vi "BRig_Host_comm_tcp_parseCmd__getType_v2.vi"(0 "input_strCmd":string, 2 "input_countCmd":i32) -> (14 "output_strType":u8)   [LabVIEW 2014]
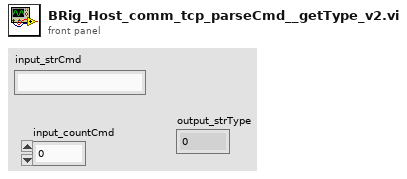
[diagram p1: front panel]
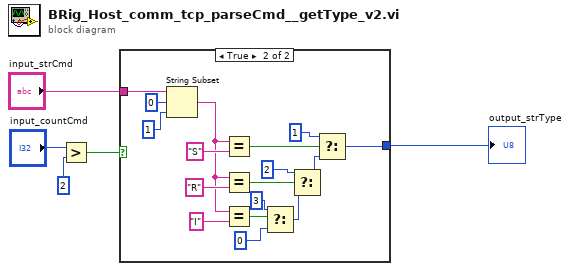
[diagram p0: block diagram]
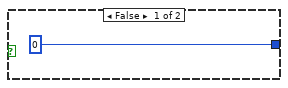
[diagram p2: hidden frame]
diagram:
  n1 = Greater?(x="input_countCmd", y=2) -> (0:w3:bool)
  n2 = case shown="True" w3 {
    tunnel: "input_strCmd" -> [_ w7]
    tunnel: [u8 0 ("t") w12] -> w2
    frame False {
    }
    frame True {
      n3 = String Subset(string=w7, offset (0)=0, length (rest)=1 ("length (rest)")) -> (substring=w8:string)
      n4 = Equal?(x=w8, y="S") -> (x = y?=w9:bool)
      n5 = Equal?(x=w8, y="R") -> (x = y?=w10:bool)
      n6 = Equal?(x=w8, y="I") -> (x = y?=w18:bool)
      n7 = Select(t=u8 3, s=w18, f=u8 0) -> (s? t:f=w15:u8)
      n8 = Select(t=u8 2, s=w10, f=w15) -> (s? t:f=w13:u8)
      n9 = Select(t=u8 1, s=w9, f=w13) -> (s? t:f=w12:u8)
    }
  }
  "output_strType" <- w2
